vi "Autonomous Mode.vi"(0 "Drive Motors":string="RobotDrive", 5 "B.Pick up":string="My Motor RefNum", 7 "A.Pick up":string="My Solenoid RefNum", 9 "Shooter":string="My Motor RefNum", 11 "Inverted Shooter":string="My Motor RefNum") -> ()   [LabVIEW 2013]
uses:
  <vilib>/Rock Robotics/WPI/Solenoid/WPI_SolenoidValue.ctl
  Auton Mode Determiner.vi
  <vilib>/Rock Robotics/WPI/RobotDrive/WPI_RobotDriveGetSetRefNum.vi
  Ultrasonic Sensor.vi
  <vilib>/Rock Robotics/WPI/RobotDrive/WPI_RobotDriveArcadeDrive_Standard(NoSaturation).vi
  <vilib>/Rock Robotics/WPI/Solenoid/Deprecated/WPI_SolenoidGetBool.vi
  <vilib>/Rock Robotics/WPI/Solenoid/WPI_SolenoidSetEnum.vi
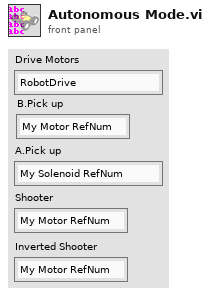
[diagram p1: front panel]
types:
  T1 = typedef "WPI_MotorControlDeviceRef.ctl" = cluster{"DeviceStatus":errorcluster, "Type":enum16{"PWM", "CAN"}, "PWM":cluster{"Digital Module":T2, "PWM Channel":T3, "DeadBand":T4}, "CAN":cluster{"Device Number":u8, "Control Mode":T5, "Semaphore":T6, "Max Vout":dbl}, "Invert":bool, "TransformRef":T7, "InvTransformRef":T7}
  T2 = typedef "FPGA_TypedefDigitalModule.ctl" = enum16{"Digital Module 1", "Digital Module 2"}
  T3 = typedef "FPGA_DIOPWMChannel.ctl" = enum8{"PWM 1", "PWM 2", "PWM 3", "PWM 4", "PWM 5", "PWM 6", "PWM 7", "PWM 8", "PWM 9", "PWM 10", "Invalid"}
  T4 = typedef "WPI_PWMDeadband.ctl" = cluster{"Name":string, "maxPositivePwm":i32, "minPositivePwm":i32, "centerPwm":i32, "maxNegativePwm":i32, "minNegativePwm":i32, "angularRange":u16}
  T5 = typedef "WPI_CANJaguar_ControlMode.ctl" = enum8{"Percent VBus", "Current", "Speed", "Position", "Voltage"}
  T6 = typedef "Semaphore RefNum" = refnum<k1>
  T7 = typedef "WPI_PWMTransform_ConPane.ctl" = refnum<vi>
  T8 = typedef "WPI_SolenoidDevRef.ctl" = cluster{"DevStatus":errorcluster, "Solenoid Module":T9, "Forward Solenoid Channel":T10, "Reverse Solenoid Channel":T10}
  T9 = typedef "FPGA_TypedefSolenoidModule.ctl" = enum16{"Solenoid Module 1", "Solenoid Module 2"}
  T10 = typedef "WPI_SolenoidChannel.ctl" = enum8{"Solenoid 1", "Solenoid 2", "Solenoid 3", "Solenoid 4", "Solenoid 5", "Solenoid 6", "Solenoid 7", "Solenoid 8", "Invalid"}
  T11 = typedef "WPI_RobotDriveDevRef.ctl" = cluster{"DevStatus":errorcluster, "Motors[]":T1[], "Square Inputs":bool, "Max Output":dbl, "Isochronous":bool}
  T12 = typedef "WPI_SolenoidValue.ctl" = enum16{"Off", "On", "Forward", "Reverse"}
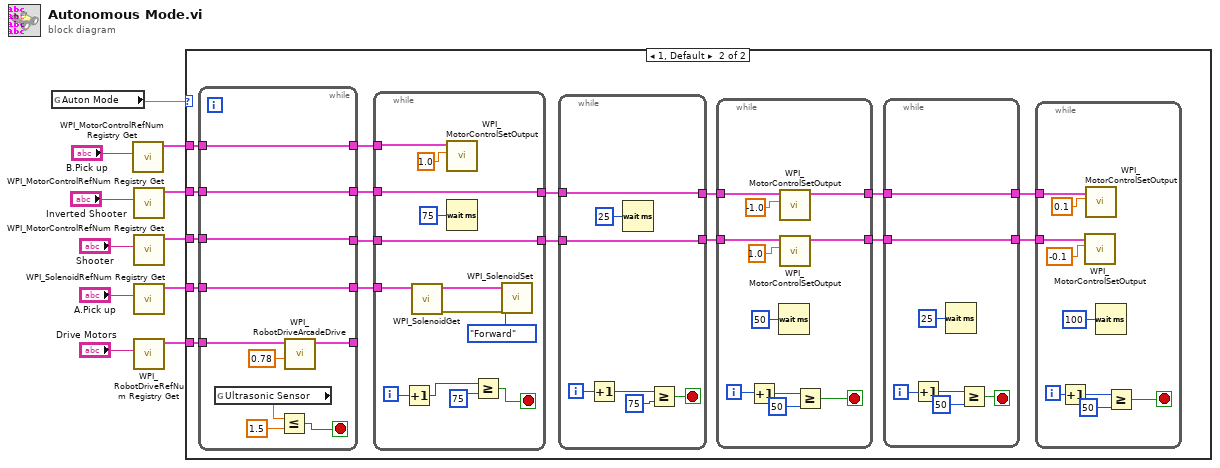
[diagram p0: block diagram]
diagram:
  n1 = global read "Auton Mode Determiner.vi" "Auton Mode"() -> (w1:dbl)
  n2 = call <vilib>:"WPI_MotorControlRefNum Registry Get.vi"("refnum name"="B.Pick up") -> ("MotorControlDevRef"=w2:T1)  [unwired: 9 in, 1 out]
  n3 = call <vilib>:"WPI_MotorControlRefNum Registry Get.vi"("refnum name"="Inverted Shooter") -> ("MotorControlDevRef"=w3:T1)  [unwired: 9 in, 1 out]
  n4 = call <vilib>:"WPI_MotorControlRefNum Registry Get.vi"("refnum name"="Shooter") -> ("MotorControlDevRef"=w4:T1)  [unwired: 9 in, 1 out]
  n5 = call <vilib>:"WPI_SolenoidRefNum Registry Get.vi"("refnum name"="A.Pick up") -> ("SolenoidDevRef"=w8:T8)  [unwired: 9 in, 1 out]
  n6 = call <vilib>:"WPI_RobotDriveRefNum Registry Get.vi"("refnum name"="Drive Motors") -> ("RobotDriveDevRef"=w11:T11)  [unwired: 9 in, 1 out]
  n7 = case shown="1, Default" w1 {
    tunnel: w11 -> [_ w28]
    tunnel: w8 -> [_ w27]
    tunnel: w4 -> [_ w26]
    tunnel: w3 -> [_ w25]
    tunnel: w2 -> [_ w24]
    frame 0 {
    }
    frame 1, Default {
      n8 = while {
        tunnel: [w85] -> _
        tunnel: w28 -> [w84]
        tunnel: w27 -> [w83]
        tunnel: [w83] -> w23
        tunnel: [w82] -> w20
        tunnel: w26 -> [w82]
        tunnel: [w81] -> w21
        tunnel: w25 -> [w81]
        tunnel: [w80] -> w22
        tunnel: w24 -> [w80]
        stop <- w77 stop-if-true
        n9 = global read "Ultrasonic Sensor.vi" "Ultrasonic Sensor"() -> (w79:dbl)
        n10 = Less Or Equal?(x=w79, y=1.5) -> (x <= y?=w77:bool)
        n11 = call-poly <vilib>:"WPI_RobotDriveArcadeDrive.vi"("Y axis value"=0.78, "RobotDriveDevRef"=w84) -> ("RobotDriveDevRef"=w85:T11)  [unwired: 7 in, 2 out]
      }
      n12 = while {
        tunnel: w23 -> [w75]
        tunnel: w22 -> [w67]
        tunnel: w21 -> [w63]
        tunnel: w20 -> [w64]
        tunnel: [w64] -> w19
        tunnel: [w63] -> w18
        i -> [w74]
        stop <- w71 stop-if-true
        n13 = Increment(x=w74) -> (x+1=w73:i32)
        n14 = call-poly <vilib>:"WPI_SolenoidGet.vi"("SolenoidDevRef"=w75) -> ("error out"=w70:errorcluster, "SolenoidDevRef"=w69:T8)  [unwired: 8 in, 1 out]
        n15 = call <vilib>:"WPI_MotorControlSetOutput.vi"("Output"=1.0, "MotorControlDevRef"=w67) -> ()  [unwired: 7 in, 3 out]
        n16 = Wait (ms)(milliseconds to wait=u32 75) -> ()  [unwired: 1 out]
        n17 = Greater Or Equal?(x=w73, y=75) -> (x >= y?=w71:bool)
        n18 = call-poly <vilib>:"WPI_SolenoidSet.vi"("error in (no error)"=w70, "Value"=WPI_SolenoidValue."Forward", "SolenoidDevRef"=w69) -> ()  [unwired: 7 in, 2 out]
      }
      n19 = while {
        tunnel: [w58] -> w17
        tunnel: w19 -> [w58]
        tunnel: w18 -> [w57]
        tunnel: [w57] -> w16
        i -> [w59]
        stop <- w60 stop-if-true
        n20 = Increment(x=w59) -> (x+1=w61:i32)
        n21 = Wait (ms)(milliseconds to wait=u32 25) -> ()  [unwired: 1 out]
        n22 = Greater Or Equal?(x=w61, y=75) -> (x >= y?=w60:bool)
      }
      n23 = while {
        tunnel: w17 -> [w50]
        tunnel: w16 -> [w51]
        tunnel: [w47] -> w15
        tunnel: [w46] -> w14
        i -> [w55]
        stop <- w52 stop-if-true
        n24 = Increment(x=w55) -> (x+1=w54:i32)
        n25 = Wait (ms)(milliseconds to wait=u32 50) -> ()  [unwired: 1 out]
        n26 = call <vilib>:"WPI_MotorControlSetOutput.vi"("Output"=-1.0, "MotorControlDevRef"=w51) -> ("MotorControlDevRef"=w46:T1)  [unwired: 7 in, 2 out]
        n27 = call <vilib>:"WPI_MotorControlSetOutput.vi"("Output"=1.0, "MotorControlDevRef"=w50) -> ("MotorControlDevRef"=w47:T1)  [unwired: 7 in, 2 out]
        n28 = Greater Or Equal?(x=w54, y=50) -> (x >= y?=w52:bool)
      }
      n29 = while {
        tunnel: w15 -> [w38]
        tunnel: w14 -> [w39]
        tunnel: [w39] -> w13
        tunnel: [w38] -> w12
        i -> [w42]
        stop <- w41 stop-if-true
        n30 = Increment(x=w42) -> (x+1=w44:i32)
        n31 = Wait (ms)(milliseconds to wait=u32 25) -> ()  [unwired: 1 out]
        n32 = Greater Or Equal?(x=w44, y=50) -> (x >= y?=w41:bool)
      }
      n33 = while {
        tunnel: w13 -> [w37]
        tunnel: w12 -> [w36]
        i -> [w33]
        stop <- w32 stop-if-true
        n34 = Increment(x=w33) -> (x+1=w34:i32)
        n35 = call <vilib>:"WPI_MotorControlSetOutput.vi"("Output"=-0.1, "MotorControlDevRef"=w36) -> ()  [unwired: 7 in, 3 out]
        n36 = call <vilib>:"WPI_MotorControlSetOutput.vi"("Output"=0.1, "MotorControlDevRef"=w37) -> ()  [unwired: 7 in, 3 out]
        n37 = Wait (ms)(milliseconds to wait=u32 100) -> ()  [unwired: 1 out]
        n38 = Greater Or Equal?(x=w34, y=50) -> (x >= y?=w32:bool)
      }
    }
  }
